vi "Host_DialogueUpdate.vi"(10 "Time in":dbl, 11 "String in":string) -> (3 "String out":string)   [LabVIEW 2017]
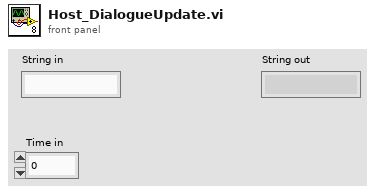
[diagram p1: front panel]
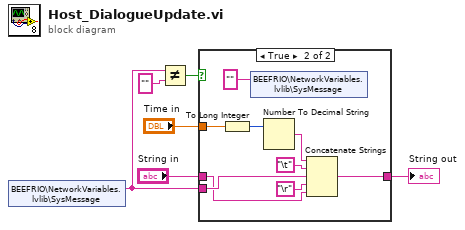
[diagram p0: block diagram]
diagram:
  n1 = shared-variable "BEEFRIO\\NetworkVariables.lvlib\\SysMessage"() -> (w2:string)  [unwired: 1 in, 1 out]
  n2 = Not Equal?(x=w2, y="" ("String")) -> (x != y?=w4:bool)
  n3 = case shown="True" w4 {
    tunnel: "String in" -> [w7 w10]
    tunnel: [w7 w9] -> w5
    tunnel: "Time in" -> [_ w14]
    tunnel: w2 -> [_ w12]
    frame False {
    }
    frame True {
      n4 = To Long Integer(number=w14) -> (32bit integer=w13:i32)
      n5 = shared-variable "BEEFRIO\\NetworkVariables.lvlib\\SysMessage"("" ("SysMessage")) -> ()  [unwired: 1 in, 1 out]
      n6 = Number To Decimal String(number=w13) -> (decimal integer string=w16:string)  [unwired: 1 in]
      n7 = Concatenate Strings(w16, "\t", w12, "\r", w10) -> (w9:string)
    }
  }
  "String out" <- w5
